vi "Flock_Shared_Wait for Valid Queue Reference.vi"(8 "error in (no error)":errorcluster, 11 "Process List":T1) -> (0 "error out":errorcluster, 2 "Numeric Control":i32, 3 "Process List Out":T1)   [LabVIEW 2013, in "Flock_Shared_Messaging.lvlib"]
uses:
  Flock_Shared_Messaging.lvlib
  ProcessList.ctl
  FGV_Action.ctl
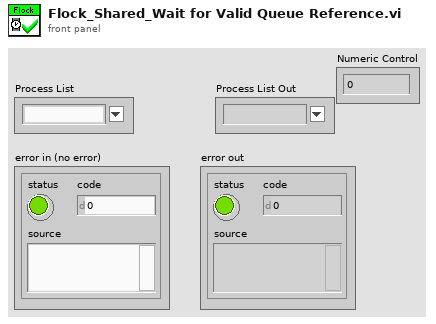
[diagram p1: front panel]
types:
  T1 = typedef "Flock_Shared_Messaging.lvlib/ProcessList.ctl" = string
  T2 = typedef "FGV_Action.ctl" = enum16{"Initalize Central", "Initialize Local", "Get", "Delete Local"}
  T3 = typedef "Flock_Shared_Messaging.lvlib/FGV_Queues.ctl" = cluster{"Local Queue in 2":T4, "Enum":T1}[]
  T4 = typedef "amc_Message Queue.ctl" = refnum<queue>
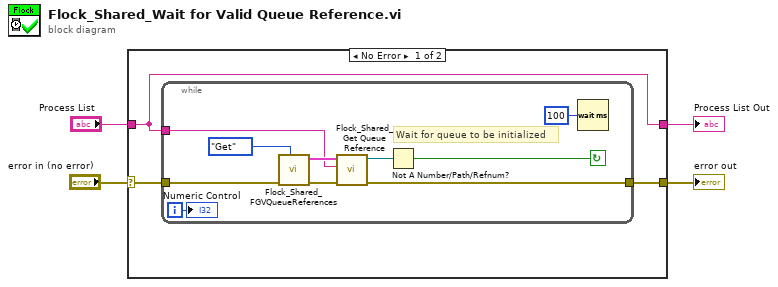
[diagram p0: block diagram]
diagram:
  n1 = case shown="No Error" "error in (no error)" {
    selector: "error in (no error)" -> [w6 w19]
    tunnel: "Process List" -> [w5 w18]
    tunnel: [w7 w19] -> w3
    tunnel: [w5 w18] -> w1
    frame No Error {
      n2 = while {
        tunnel: [w17] -> w7
        tunnel: w5 -> [w8]
        tunnel: w6 -> [w14]
        i -> [w10]
        stop <- w12 continue-if-true
        # "Wait for queue to be initialized"
        n3 = call "Flock_Shared_FGVQueueReferences.vi"("Action"=FGV_Action."Get", "error in (no error)"=w14) -> ("error out"=w13:errorcluster, "Array"=w16:T3)  [unwired: 7 in, 1 out]
        n4 = call "Flock_Shared_Get Queue Reference.vi"("Error In"=w13, "Enum"=w8, "Array"=w16) -> ("Error Out"=w17:errorcluster, "Local Queue out"=w11:T4)  [unwired: 7 in]
        n5 = Not A Number/Path/Refnum?(number/path/refnum=w11) -> (NaN/Path/Refnum?=w12:bool)
        n6 = Wait (ms)(milliseconds to wait=u32 100) -> ()  [unwired: 1 out]
        "Numeric Control" <- w10
      }
    }
    frame Error {
    }
  }
  "error out" <- w3
  "Process List Out" <- w1
